vi "Astar on Occupancy Grid.vi"(7 "goal node":cluster{"X":i32, "Y":i32}={"X"=0, "Y"=6}, 8 "start node":cluster{"X":i32, "Y":i32}, 9 "roadBlocks":bool[][](array[boolean])) -> (0 "Intensity Graph 2":dbl[][](graph)=[[50.0, 100.0, 50.0, 50.0, 50.0, 50.0, 0.0], [50.0, 100.0, 50.0, 100.0, 100.0, 100.0, 1.0], [50.0, 100.0, 50.0, 50.0, 50.0, 100.0, 1.0], [50.0, 100.0, 100.0, 100.0, 50.0, 100.0, 100.0], [50.0, 50.0, 50.0, 50.0, 50.0, 1.0, 1.0]] caption="Intensity Graph", 2 "y":i32[](array[numeric])=[0, 1, 2, 2, 2, 1, 1, 0, 0, 0], 3 "x":i32[](array[numeric])=[0, 0, 0, 1, 2, 2, 1, 1, 2, 3])   [LabVIEW 2016]
doc: "This example shows how to use the A* algorithm with an occupancy grid to compute the shortest path between start and goal nodes."
uses:
  <vilib>/Utility/miscctls.llb/LVPoint32TypeDef.ctl
  <vilib>/robotics/Navigation/shared/WorldMap/OccupancyGridWorldMap/NI_Robotics_OccupancyGridWorldMap.lvclass
panel:
  out "String":string="right"
  out "Numeric":i32
  out "i":i32=17
  out "filledcorners":dbl[][](array[numeric])=[[-2.0, 100.0, -2.0, -2.0, -2.0, -2.0, -2.0], [-2.0, 100.0, -2.0, 100.0, 100.0, 100.0, 1.0], [-2.0, 100.0, -2.0, -2.0, -2.0, 100.0, 1.0], [-2.0, 100.0, 100.0, 100.0, -2.0, 100.0, 100.0], [-2.0, -2.0, -2.0, -2.0, -2.0, 1.0, 1.0]]
  out "Array out":bool[][](array[boolean])=[[TRUE, FALSE, TRUE, TRUE, TRUE, TRUE, TRUE], [TRUE, FALSE, TRUE, FALSE, FALSE, FALSE, FALSE], [TRUE, FALSE, TRUE, TRUE, TRUE, FALSE, FALSE], [TRUE, FALSE, FALSE, FALSE, TRUE, FALSE, FALSE], [TRUE, TRUE, TRUE, TRUE, TRUE, FALSE, FALSE]]
  out "Path":bool[][](array[boolean])=[[TRUE, FALSE, TRUE, FALSE, FALSE, FALSE, TRUE], [FALSE, FALSE, FALSE, FALSE, FALSE, FALSE, FALSE], [FALSE, FALSE, TRUE, FALSE, TRUE, FALSE, FALSE], [FALSE, FALSE, FALSE, FALSE, FALSE, FALSE, FALSE], [TRUE, FALSE, FALSE, FALSE, TRUE, FALSE, FALSE]]
  out "intensity values":dbl[][](array[numeric])=[[-2.0, 100.0, 1.0, -2.0, -2.0, -2.0, -2.0], [-2.0, 100.0, -2.0, 100.0, 100.0, 100.0, 1.0], [-2.0, 100.0, 1.0, -2.0, 1.0, 100.0, 1.0], [-2.0, 100.0, 100.0, 100.0, -2.0, 100.0, 100.0], [1.0, -2.0, -2.0, -2.0, 1.0, 1.0, 1.0]]
  out "Array 2":i32[][](array[numeric])=[[1, 100, 1, 1, 1, 1, 1], [1, 100, 1, 100, 100, 100, 1], [1, 100, 1, 1, 1, 100, 1], [1, 100, 100, 100, 1, 100, 100], [1, 1, 1, 1, 1, 1, 1]]
  in  "Action":enum32{"Mark Obstacle", "Set Start", "Set Goal"}(radio)
  out "Intensity Graph":dbl[][](graph)=[[-2.0, 100.0, 1.0, -2.0, -2.0, -2.0, -2.0], [-2.0, 100.0, -2.0, 100.0, 100.0, 100.0, 1.0], [-2.0, 100.0, 1.0, -2.0, 1.0, 100.0, 1.0], [-2.0, 100.0, 100.0, 100.0, -2.0, 100.0, 100.0], [1.0, -2.0, -2.0, -2.0, 1.0, 1.0, 1.0]]
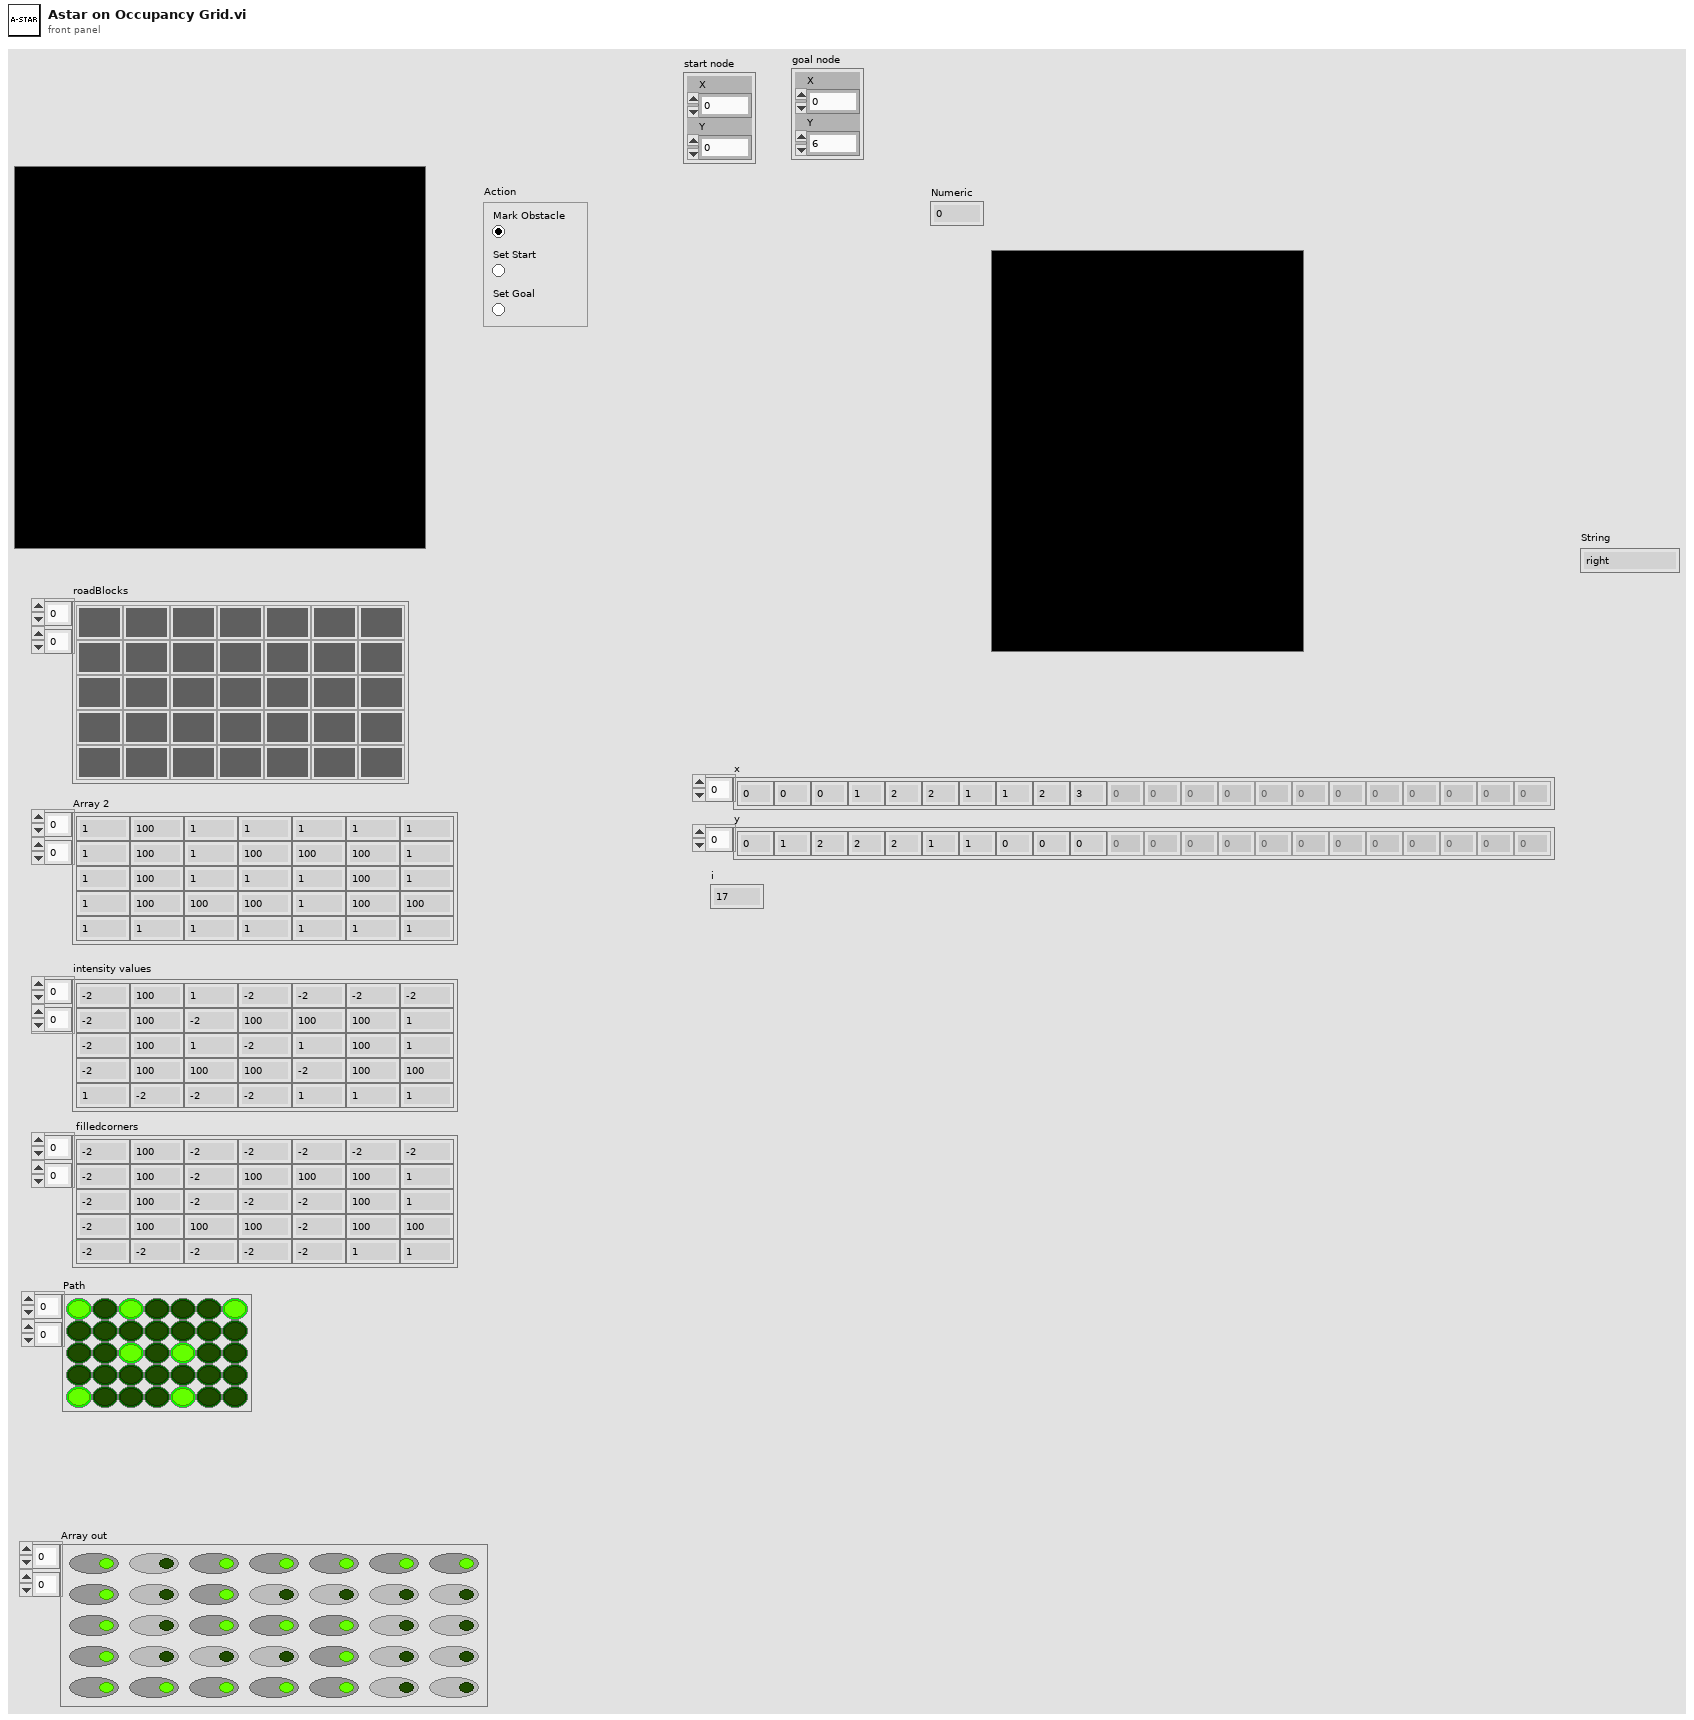
[diagram p1: front panel]
types:
  T1 = typedef "LVPoint32TypeDef.ctl" = cluster{"Horizontal":i32, "Vertical":i32}
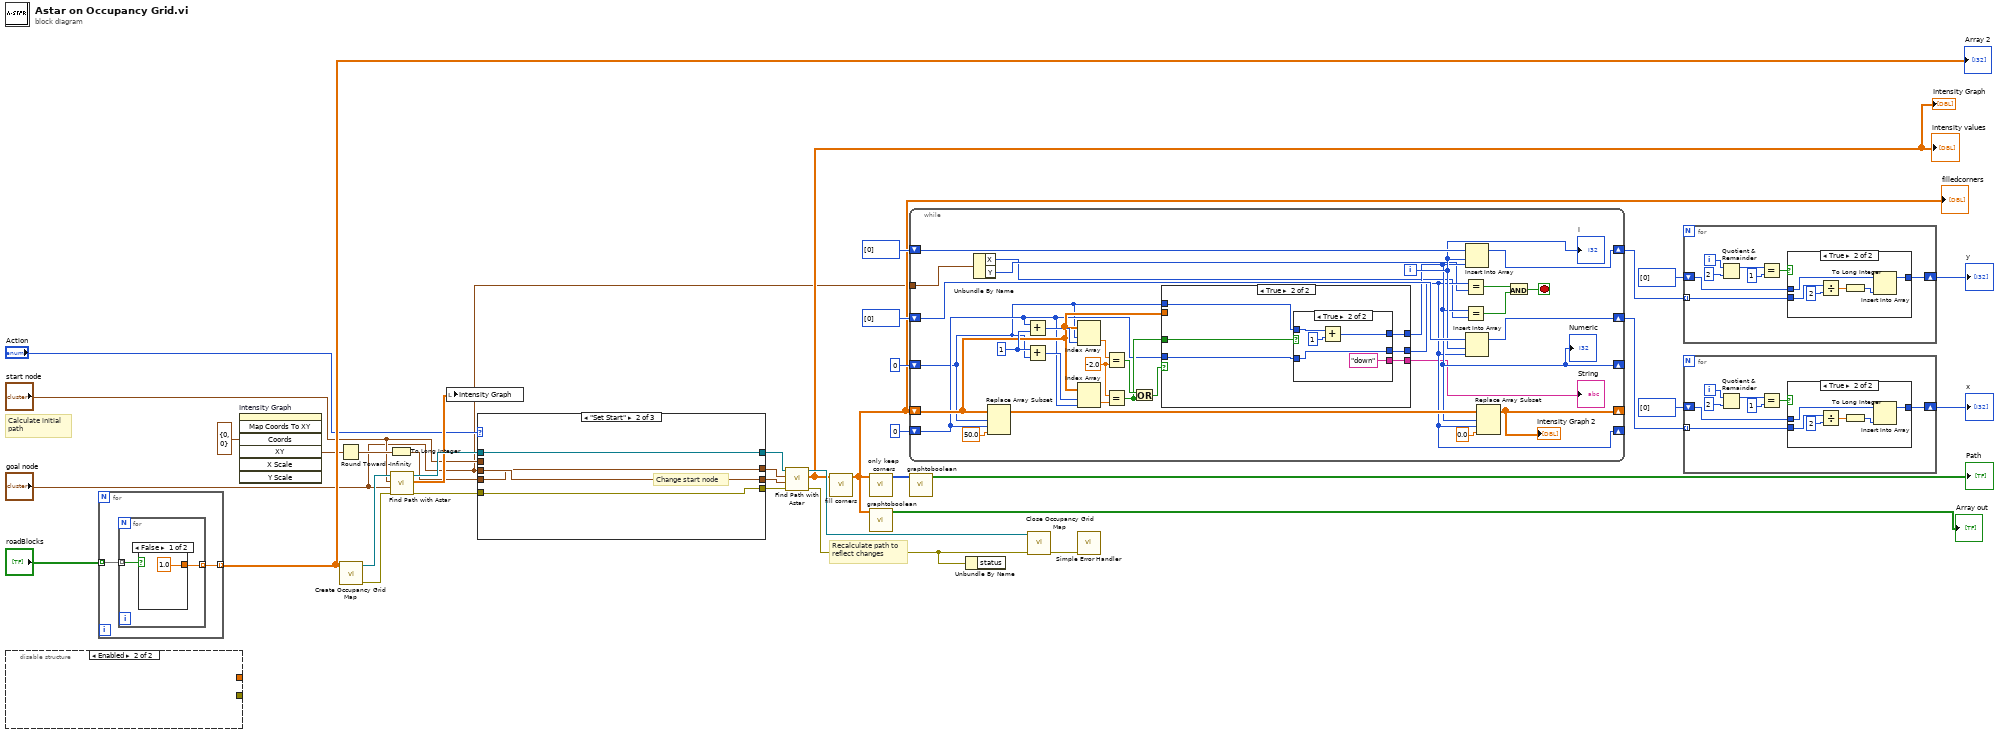
[diagram p0: block diagram]
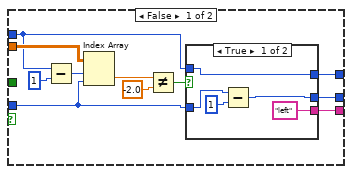
[diagram p4: hidden frame]
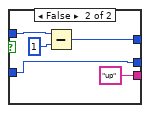
[diagram p5: hidden frame]
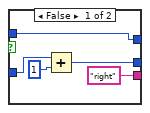
[diagram p6: hidden frame]
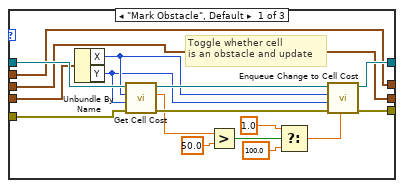
[diagram p7: hidden frame]
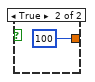
[diagram p9: hidden frame]
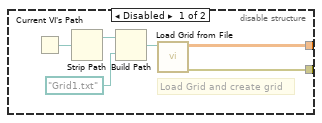
[diagram p10: hidden frame]
diagram:
  # "Recalculate path to\nreflect changes"
  # "Calculate initial \npath"
  n1 = disable-structure shown="Enabled" {
    disable-tunnel: [w38 _] -> _
    disable-tunnel: [w37 _] -> _
    frame Disabled {
      # "Load Grid and create grid"
      n2 = Current VI's Path() -> (path=w42:path)
      n3 = Strip Path(path=w42) -> (stripped path=w41:path)  [unwired: 1 out]
      n4 = Build Path(base path=w41, name or relative path=path "Grid1.txt" ("stripped path")) -> (appended path=w39:path)
      n5 = call "Load Grid from File.vi"("file path"=w39) -> ("error out"=w37:errorcluster, "occupancy grid"=w38:dbl[][])  [unwired: 8 in, 1 out]
    }
    frame Enabled {
    }
  }
  n6 = for {
    tunnel: "roadBlocks" -> [w44] mode=indexing
    tunnel: [w43] -> w28 mode=indexing
    n7 = for {
      tunnel: w44 -> [w46] mode=indexing
      tunnel: [w45] -> w43 mode=indexing
      n8 = case shown="False" w46 {
        tunnel: [1.0 100] -> w45
        frame False {
        }
        frame True {
        }
      }
    }
  }
  "Array 2" <- w28
  n9 = invoke on="Intensity Graph" class="IntGraph (strict)" method="Map Coords To XY"("Coords"=T1 {"Horizontal"=0, "Vertical"=0}) -> ("XY"=w25:cluster{"X":dbl, "Y":dbl})  [unwired: 6 in, 6 out]
  n10 = Round Toward -Infinity(1:w25) -> (0:w24:cluster{"X":dbl, "Y":dbl})
  n11 = call <vilib>:"Create Occupancy Grid Map.vi"("occupancy grid"=w28) -> ("error out"=w31:errorcluster, "map reference out"=w33:refnum<data-value>)  [unwired: 9 in]
  n12 = To Long Integer(number=w24) -> (32bit integer=w22:cluster{"X":i32, "Y":i32})
  n13 = call "Find Path with Astar.vi"("error in (no error)"=w31, "goal node"="goal node", "start node"="start node", "map reference in"=w33) -> ("error out"=w30:errorcluster, "intensity values"=w29:dbl[][], "map reference out"=w32:refnum<data-value>)  [unwired: 5 in]
  n14 = local write "Intensity Graph"(w29) -> ()
  n15 = case shown="\"Set Start\"" "Action" {
    tunnel: w32 -> [w65 w67 w71]
    tunnel: w30 -> [w63 w66 w70]
    tunnel: [w55 w66 w70] -> w20
    tunnel: [w54 w67 w71] -> w21
    tunnel: "start node" -> [w53 _ w73]
    tunnel: "goal node" -> [w52 w69 _]
    tunnel: [w53 w68 w73] -> w27
    tunnel: [w52 w69 w72] -> w26
    tunnel: w22 -> [w49 w68 w72]
    frame "Mark Obstacle", Default {
      # "Toggle whether cell\nis an obstacle and update"
      n16 = Unbundle By Name(w49) -> ("X"=w51:i32, "Y"=w50:i32)
      n17 = call <vilib>:"Get Cell Cost.vi"("error in (no error)"=w63, "y"=w50, "x"=w51, "map reference in"=w65) -> ("error out"=w62:errorcluster, "cost"=w61:dbl, "map reference out"=w64:refnum<data-value>)  [unwired: 4 in, 1 out]
      n18 = Greater?(x=w61, y=50.0) -> (0:w59:bool)
      n19 = Select(t=1.0, s=w59, f=100.0) -> (s? t:f=w56:dbl)
      n20 = call <vilib>:"Enqueue Change to Cell Cost.vi"("cost"=w56, "error in (no error)"=w62, "y"=w50, "x"=w51, "map reference in"=w64) -> ("error out"=w55:errorcluster, "map reference out"=w54:refnum<data-value>)  [unwired: 5 in]
    }
    frame "Set Start" {
      # "Change start node"
    }
    frame "Set Goal" {
      # "change goal node"
    }
  }
  n21 = call "Find Path with Astar.vi"("error in (no error)"=w20, "goal node"=w26, "start node"=w27, "map reference in"=w21) -> ("error out"=w36:errorcluster, "intensity values"=w19:dbl[][], "map reference out"=w34:refnum<data-value>)  [unwired: 5 in]
  "Intensity Graph" <- w19
  "intensity values" <- w19
  n22 = call "fill corners.vi"("intensity values"=w19) -> ("Array"=w10:dbl[][])  [unwired: 10 in]
  "filledcorners" <- w10
  n23 = call "only keep corners.vi"("intensity values"=w10) -> ("Array"=w17:i32[][])  [unwired: 10 in]
  n24 = call "graphtoboolean.vi"("Array in"=w10) -> ("Array out"=→"Array out":bool[][])  [unwired: 10 in]
  n25 = while {
    shift-right: [w87] -> w6
    shift-left: i32[] [0] -> [w103]
    shift-right: [w79] -> _
    shift-left: 0 -> [w84]
    shift-right: [w80] -> _
    shift-left: 0 -> [w83]
    shift-right: [w86] -> w8
    shift-left: i32[] [0] -> [w99]
    shift-right: [w81] -> _
    shift-left: w10 -> [w88]
    tunnel: "goal node" -> [w76]
    i -> [w98]
    stop <- w102 stop-if-true
    w94 = -2.0 ("x")
    w97 = 1 ("y")
    n26 = Unbundle By Name(w76) -> ("X"=w74:i32, "Y"=w75:i32)
    n27 = Replace Array Subset(array=w88, new element=50.0 ("new element/subarray"), index (row)=w83, index (col)=w84) -> (w82:dbl[][])
    n28 = Add(x=w84, y=w97) -> (x+y=w90:i32)
    n29 = Add(x=w97, y=w83) -> (x+y=w89:i32)
    n30 = Index Array(array=w88, index (row)=w83, index (col)=w90) -> (element=w96:dbl)
    n31 = Index Array(array=w88, index (row)=w89, index (col)=w84) -> (element=w95:dbl)
    n32 = Equal?(x=w96, y=w94) -> (x = y?=w93:bool)
    n33 = Equal?(x=w94, y=w95) -> (x = y?=w91:bool)
    n34 = Or(x=w93, y=w91) -> (x .or. y?=w92:bool)
    n35 = case shown="True" w92 {
      tunnel: w84 -> [w104 w127]
      tunnel: w83 -> [w107 w129]
      tunnel: w91 -> [_ w130]
      tunnel: [w114 w128] -> w79
      tunnel: [w113 w126] -> w80
      tunnel: w88 -> [w109 _]
      tunnel: [w106 w125] -> w77
      frame False {
        n36 = Subtract(x=w107, y=1) -> (x-y=w105:i32)
        n37 = Index Array(array=w109, index (row)=w105, index (col)=w104) -> (element=w111:dbl)
        n38 = Not Equal?(x=w111, y=-2.0 ("x")) -> (x != y?=w108:bool)
        n39 = case shown="True" w108 {
          tunnel: w107 -> [w116 w124]
          tunnel: [w117 w122] -> w114
          tunnel: w104 -> [w118 w122]
          tunnel: [w116 w121] -> w113
          tunnel: ["left" ("String") "up" ("String")] -> w106
          frame True {
            n40 = Subtract(x=w118, y=1) -> (x-y=w117:i32)
          }
          frame False {
            n41 = Subtract(x=w124, y=1) -> (x-y=w121:i32)
          }
        }
      }
      frame True {
        n42 = case shown="True" w130 {
          tunnel: w129 -> [w132 w140]
          tunnel: [w133 w138] -> w128
          tunnel: w127 -> [w134 w138]
          tunnel: [w132 w137] -> w126
          tunnel: ["right" ("String") "down" ("String")] -> w125
          frame False {
            n43 = Add(x=w134, y=1) -> (x+y=w133:i32)
          }
          frame True {
            n44 = Add(x=w140, y=1) -> (x+y=w137:i32)
          }
        }
      }
    }
    "Numeric" <- w80
    "String" <- w77
    n45 = Equal?(x=w79, y=w75) -> (x = y?=w101:bool)
    n46 = Equal?(x=w80, y=w74) -> (x = y?=w100:bool)
    n47 = Insert Into Array(array=w103, index=w98, new element=w80) -> (w87:i32[])
    n48 = Insert Into Array(array=w99, index=w98, new element=w79) -> (w86:i32[])
    n49 = Replace Array Subset(array=w82, new element=0.0 ("new element/subarray"), index (row)=w80, index (col)=w79) -> (w81:dbl[][])
    "Intensity Graph 2" <- w81
    n50 = And(x=w101, y=w100) -> (x .and. y?=w102:bool)
    "i" <- w98
  }
  n51 = call "graphtoboolean.vi"("Array in"=w17) -> ("Array out"=→"Path":bool[][])  [unwired: 10 in]
  n52 = Unbundle By Name(w36) -> ()  [unwired: 1 out]
  n53 = call <vilib>:"Close Occupancy Grid Map.vi"("error in (no error)"=w36, "map reference in"=w34) -> ("error out"=w35:errorcluster)  [unwired: 9 in]
  n54 = call <vilib>:"Simple Error Handler.vi"("error in (no error)"=w35) -> ()  [unwired: 4 in, 5 out]
  n55 = for {
    shift-right: [w143] -> w5
    shift-left: i32[] [0] -> [w144]
    tunnel: w6 -> [w142] mode=indexing
    i -> [w141]
    n56 = Quotient & Remainder(x=w141, y=2) -> (x-y*floor(x/y)=w147:i32)  [unwired: 1 out]
    n57 = Equal?(x=w147, y=1) -> (x = y?=w145:bool)
    n58 = case shown="True" w145 {
      tunnel: w144 -> [w149 w155]
      tunnel: [w149 w154] -> w143
      tunnel: w142 -> [_ w153]
      frame False {
      }
      frame True {
        n59 = Divide(x=w153, y=2) -> (x/y=w151:dbl)
        n60 = To Long Integer(number=w151) -> (32bit integer=w150:i32)
        n61 = Insert Into Array(array=w155, new element=w150) -> (w154:i32[])  [unwired: 1 in]
      }
    }
  }
  "y" <- w5
  n62 = for {
    shift-right: [w158] -> w4
    shift-left: i32[] [0] -> [w159]
    tunnel: w8 -> [w157] mode=indexing
    i -> [w156]
    n63 = Quotient & Remainder(x=w156, y=2) -> (x-y*floor(x/y)=w162:i32)  [unwired: 1 out]
    n64 = Equal?(x=w162, y=1) -> (x = y?=w160:bool)
    n65 = case shown="True" w160 {
      tunnel: w159 -> [w164 w170]
      tunnel: [w164 w169] -> w158
      tunnel: w157 -> [_ w167]
      frame False {
      }
      frame True {
        n66 = Divide(x=w167, y=2) -> (x/y=w166:dbl)
        n67 = To Long Integer(number=w166) -> (32bit integer=w165:i32)
        n68 = Insert Into Array(array=w170, new element=w165) -> (w169:i32[])  [unwired: 1 in]
      }
    }
  }
  "x" <- w4
